vi "Read CSM Status with lvcsm Support.vi"(6 "Config Path (\"\" For Lvcsm File)":path, 7 "Current Module (\"\" to Generate an ID)":string, 8 "error in (no error)":errorcluster, 9 "Force? (F)":bool, 11 "CSM Name":string) -> (0 "error out":errorcluster, 3 "CSMAPI List":string[](array[string]))   [LabVIEW 2017, in "CSM-Helper API with lvcsm Support.lvlib"]
uses:
  CSM-Helper API with lvcsm Support.lvlib
  _Read CSM Status Content.vi
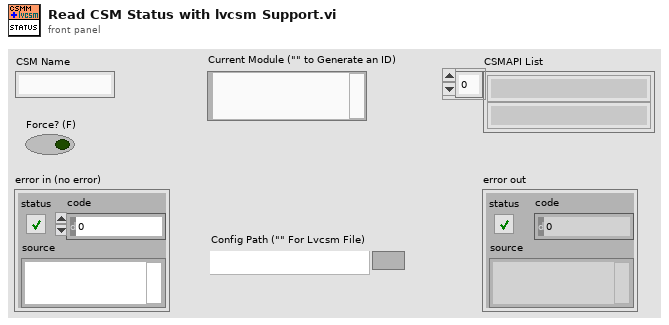
[diagram p1: front panel]
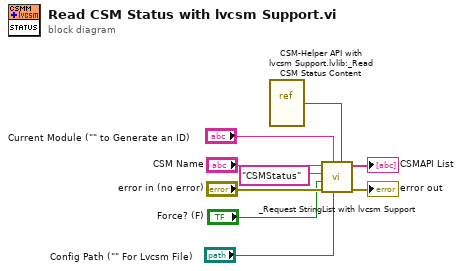
[diagram p0: block diagram]
diagram:
  n1 = vi-ref "CSM-Helper API with lvcsm Support.lvlib:_Read CSM Status Content.vi"() -> (w2:refnum<vi>)
  n2 = call "_Request StringList with lvcsm Support.vi"("API Ref"=w2, "Config Path (\"\" For Lvcsm File)"="Config Path (\"\" For Lvcsm File)", "Current Module (\"\" to Generate an ID)"="Current Module (\"\" to Generate an ID)", "error in (no error)"="error in (no error)", "Force? (F)"="Force? (F)", "API Name"="CSMStatus", "CSM Name"="CSM Name") -> ("error out"=→"error out":errorcluster, "CSMAPI List"=→"CSMAPI List":string[])  [unwired: 3 in]
